vi "Test Q factor retrieval.vi"() -> ()   [LabVIEW 2012]
uses:
  Reusable/General/Math Utilities.lvlib
  <vilib>/Analysis/NI_AALBase.lvlib
  <vilib>/Analysis/baseanly.llb/Mean (DBL).vi
panel:
  out "Waveform Graph":dbl[][](graph)
  out "element":timestamp
  in  "Cell":i32
  out "Q with offset":dbl
  out "best fit parameters 2":dbl[](array[numeric])
  out "Q Factor 2":dbl
  in  "index":i32 min=0 max=1000
  out "prev Qfactor":dbl
  out "Q Factor":dbl
  out "best fit parameters":dbl[](array[numeric])
  in  "high":i32
  in  "low":i32
  out "XY Graph":cluster{i32[], "best fit parameters":dbl[]}[](graph)
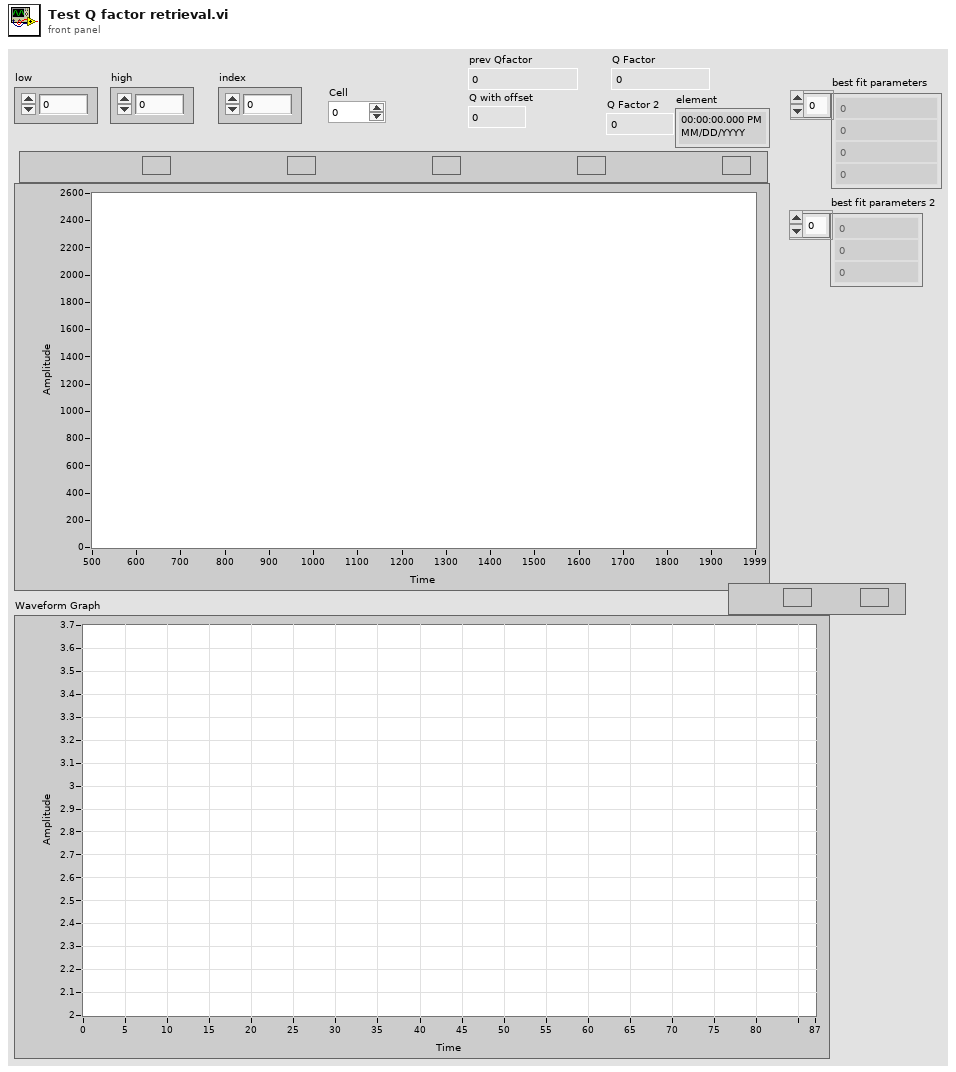
[diagram p1: front panel]
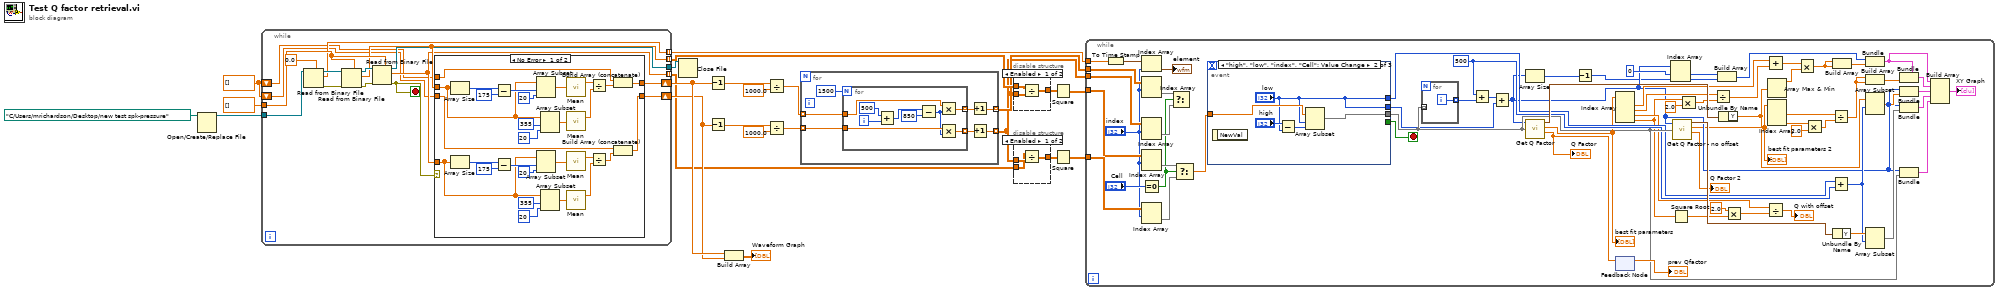
[diagram p0: block diagram]
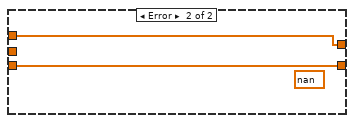
[diagram p4: hidden frame]
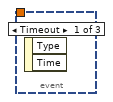
[diagram p5: hidden frame]
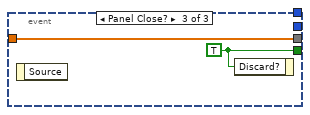
[diagram p6: hidden frame]
diagram:
  w18 = dbl[] []
  n1 = Open/Create/Replace File(file path (use dialog)=path "C:/Users/mrichardson/Desktop/new test spk-pressure") -> (refnum out=w23:refnum<file>)  [unwired: 5 in, 2 out]
  n2 = while {
    tunnel: w23 -> [w32]
    tunnel: dbl[] [] -> [w36]
    tunnel: [w39] -> w21
    tunnel: [w29] -> w1 mode=indexing
    tunnel: [w30] -> w6 mode=indexing
    tunnel: [w31] -> w19 mode=indexing
    shift-right: [w27] -> w16
    shift-left: w18 -> [w25]
    shift-right: [w26] -> w10
    shift-left: w18 -> [w24]
    stop <- w28 stop-if-true
    n3 = Read from Binary File(5:0.0, 11:w32) -> (0:w33:errorcluster, 2:w31:dbl, 3:w34:refnum<file>)  [unwired: 4 in, 1 out]
    n4 = Read from Binary File(5:w36, 8:w33, 11:w34) -> (0:w38:errorcluster, 2:w30:dbl[], 3:w37:refnum<file>)  [unwired: 3 in, 1 out]
    n5 = Read from Binary File(5:w36, 8:w38, 11:w37) -> (0:w28:errorcluster, 2:w29:dbl[], 3:w39:refnum<file>)  [unwired: 3 in, 1 out]
    n6 = case shown="No Error" w28 {
      tunnel: w30 -> [w63 _]
      tunnel: w29 -> [w41 _]
      tunnel: [w46 w69] -> w27
      tunnel: [w44 w68] -> w26
      tunnel: w25 -> [w43 w69]
      tunnel: w24 -> [w42 w68]
      frame No Error {
        n7 = Array Size(array=w63) -> (size(s)=w67:i32)
        n8 = Array Size(array=w41) -> (size(s)=w57:i32)
        n9 = Subtract(x=w67, y=175) -> (x-y=w65:i32)
        n10 = Subtract(x=w57, y=175) -> (x-y=w55:i32)
        n11 = Array Subset(array=w63, index=w65, length=20) -> (w59:dbl[])
        n12 = Array Subset(array=w41, index=w55, length=20) -> (w48:dbl[])
        n13 = Array Subset(array=w63, index=355, length=20) -> (w60:dbl[])
        n14 = Array Subset(array=w41, index=355, length=20) -> (w51:dbl[])
        n15 = call-poly <vilib>:"Mean.vi"("X"=w59) -> ("mean"=w40:dbl)  [unwired: 1 out]
        n16 = call-poly <vilib>:"Mean.vi"("X"=w60) -> ("mean"=w58:dbl)  [unwired: 1 out]
        n17 = call-poly <vilib>:"Mean.vi"("X"=w48) -> ("mean"=w50:dbl)  [unwired: 1 out]
        n18 = call-poly <vilib>:"Mean.vi"("X"=w51) -> ("mean"=w49:dbl)  [unwired: 1 out]
        n19 = Divide(x=w40, y=w58) -> (x/y=w47:dbl)
        n20 = Divide(x=w50, y=w49) -> (x/y=w45:dbl)
        n21 = Build Array (concatenate)(w43, w47) -> (w46:dbl[])
        n22 = Build Array (concatenate)(w42, w45) -> (w44:dbl[])
      }
      frame Error {
        (unwired) nan ("mean")
      }
    }
  }
  n23 = Close File(refnum=w21) -> ()  [unwired: 1 in, 2 out]
  n24 = Decrement(x=w16) -> (x-1=w15:dbl[])
  n25 = Decrement(x=w10) -> (x-1=w9:dbl[])
  n26 = Build Array(w16, w10) -> (→"Waveform Graph":dbl[][])
  n27 = Divide(x=w15, y=1000.0) -> (x/y=w12:dbl[])
  n28 = Divide(x=w9, y=1000.0) -> (x/y=w11:dbl[])
  n29 = for {
    tunnel: w12 -> [w75] mode=indexing
    tunnel: w11 -> [w76] mode=indexing
    tunnel: [w73] -> w4 mode=indexing
    tunnel: [w71] -> w3 mode=indexing
    n30 = for {
      N: 1500 -> [_]
      tunnel: w76 -> [w85]
      tunnel: w75 -> [w84]
      tunnel: [w83] -> w74 mode=indexing
      tunnel: [w82] -> w72 mode=indexing
      i -> [w81]
      n31 = Add(x=500, y=w81) -> (x+y=w79:i32)
      n32 = Subtract(x=w79, y=850) -> (x-y=w77:i32)
      n33 = Multiply(x=w84, y=w77) -> (x*y=w83:dbl)
      n34 = Multiply(x=w85, y=w77) -> (x*y=w82:dbl)
    }
    n35 = Increment(x=w74) -> (x+1=w73:dbl[])
    n36 = Increment(x=w72) -> (x+1=w71:dbl[])
  }
  n37 = disable-structure shown="Enabled" {
    disable-tunnel: w6 -> [w88 w89]
    disable-tunnel: [w87 w89] -> w5
    disable-tunnel: w4 -> [w86 _]
    frame Enabled {
      n38 = Divide(x=w88, y=w86) -> (x/y=w87:dbl[][])
    }
    frame Disabled {
    }
  }
  n39 = disable-structure shown="Enabled" {
    disable-tunnel: w3 -> [w92 _]
    disable-tunnel: w1 -> [w91 w93]
    disable-tunnel: [w90 w93] -> w2
    frame Enabled {
      n40 = Divide(x=w91, y=w92) -> (x/y=w90:dbl[][])
    }
    frame Disabled {
    }
  }
  n41 = Square(x=w5) -> (x^2=w8:dbl[][])
  n42 = Square(x=w2) -> (x^2=w7:dbl[][])
  n43 = while {
    tunnel: w7 -> [w153]
    tunnel: w8 -> [w107]
    tunnel: w19 -> [w103]
    tunnel: w4 -> [w100]
    tunnel: w3 -> [w99]
    stop <- w161 stop-if-true
    w145 = 500
    n44 = To Time Stamp(1:w103) -> (0:w102:timestamp[])
    n45 = Index Array(array=w102, index="index") -> (element=→"element":timestamp)
    n46 = Index Array(array=w100, index (row)="index") -> (element=w96:dbl[])  [unwired: 1 in]
    n47 = Index Array(array=w99, index (row)="index") -> (element=w97:dbl[])  [unwired: 1 in]
    n48 = Index Array(array=w107, index (row)="index") -> (element=w105:dbl[])  [unwired: 1 in]
    n49 = Equal To 0?(x="Cell") -> (x = 0?=w95:bool)
    n50 = Index Array(array=w153, index (row)="index") -> (element=w104:dbl[])  [unwired: 1 in]
    n51 = Select(t=w96, s=w95, f=w97) -> ()  [unwired: 1 out]
    n52 = Select(t=w105, s=w95, f=w104) -> (s? t:f=w94:dbl[])
    n53 = event shown="[1] \"high\", \"low\", \"index\", \"Cell\": Value Change" {
      selector: _ -> [_ _ _]
      dyn-events: _ -> [_ _ _]
      timeout: _ -> [_ _ _]
      tunnel: [_ _ w168] -> w161
      tunnel: w94 -> [_ w166 w169]
      tunnel: [_ w165 w169] -> w152
      tunnel: [_ "low" _] -> w146
      tunnel: [_ "low" _] -> w144
      event Timeout {
        n54 = event-data() -> ()  [unwired: 1 in, 2 out]
      }
      event "high", "low", "index", "Cell": Value Change {
        n55 = event-data() -> ()  [unwired: 1 in, 1 out]
        n56 = Subtract(x="high", y="low") -> (x-y=w164:i32)
        n57 = Array Subset(array=w166, index="low", length=w164) -> (w165:dbl[])
      }
      event Panel Close? {
        w168 = TRUE
        n58 = event-data() -> ()  [unwired: 1 in, 1 out]
        n59 = event-data("Discard?"=w168) -> ()  [unwired: 1 in, 1 out]
      }
    }
    n60 = for {
      tunnel: w152 -> [_] mode=indexing
      tunnel: [w162] -> w157 mode=indexing
      i -> [w162]
    }
    n61 = Add(x=w145, y=w157) -> (x+y=w147:i32[])
    n62 = Add(x=w147, y=w146) -> (x+y=w127:i32[])
    n63 = Array Size(array=w127) -> (size(s)=w126:i32)
    n64 = call "Get Q Factor.vi"("X"=w127, "Y"=w152) -> ("Fitted Data"=w160:waveform(dbl), "best fit parameters"=w142:dbl[], "Q Factor"=w159:dbl)  [unwired: 1 in, 2 out]
    "best fit parameters" <- w142
    "Q Factor" <- w159
    n65 = Decrement(x=w126) -> (x-1=w125:i32)
    n66 = Index Array(array=w142) -> (element #1=w129:dbl, element #2=w134:dbl, element #3=w138:dbl, element #4=w133:dbl)  [unwired: 4 in]
    n67 = feedback-in #1(w159) -> ()
    n68 = feedback #1() -> (→"prev Qfactor":dbl)  [unwired: 1 in]
    n69 = Index Array(array=w127, index #1=0 ("index"), index #2=w125) -> (element #1=w124:i32, element #2=w123:i32)
    n70 = Square Root(x=w133) -> (sqrt(x)=w141:dbl)
    n71 = call "Get Q Factor - no offset.vi"("X"=w127, "Y"=w152) -> ("Fitted Data"=w151:waveform(dbl), "best fit parameters"=w120:dbl[], "Q Factor"=→"Q Factor 2":dbl)  [unwired: 1 in, 2 out]
    "best fit parameters 2" <- w120
    n72 = Multiply(x=w133, y=2.0) -> (x*y=w131:dbl)
    n73 = Divide(x=w134, y=w131) -> (x/y=w130:dbl)
    n74 = Build Array(w124, w123) -> (w122:i32[])
    n75 = Unbundle By Name(w160) -> ("Y"=w111:dbl[])
    n76 = Multiply(x=2.0, y=w141) -> (x*y=w139:dbl)
    n77 = Add(x=w129, y=w130) -> (x+y=w110:dbl)
    n78 = Divide(x=w138, y=w139) -> (x/y=→"Q with offset":dbl)
    n79 = Array Max & Min(array=w111) -> (max value=w109:dbl)  [unwired: 3 out]
    n80 = Index Array(array=w120) -> (element #1=w116:dbl, element #3=w118:dbl)  [unwired: 3 in, 1 out]
    n81 = Multiply(x=w110, y=w109) -> (x*y=w108:dbl)
    n82 = Multiply(x=w118, y=2.0) -> (x*y=w117:dbl)
    n83 = Divide(x=w116, y=w117) -> (x/y=w115:dbl)
    n84 = Add(x=w144, y=w145) -> (x+y=w143:i32)
    n85 = Build Array(w108, w108) -> (w121:dbl[])
    n86 = Unbundle By Name(w151) -> ("Y"=w150:dbl[])
    n87 = Bundle(w122, w121) -> (w113:cluster{i32[], dbl[]})  [unwired: 1 in]
    n88 = Build Array(w115, w115) -> (w114:dbl[])
    n89 = Array Subset(array=w111, index=w143) -> (w154:dbl[])  [unwired: 1 in]
    n90 = Array Subset(array=w150, index=w143) -> (w149:dbl[])  [unwired: 1 in]
    n91 = Bundle(cluster=w113, w114) -> (w112:cluster{i32[], dbl[]})  [unwired: 1 in]
    n92 = Bundle(w127, w154) -> (w156:cluster{i32[], dbl[]})  [unwired: 1 in]
    n93 = Bundle(w127, w149) -> (w135:cluster{i32[], dbl[]})  [unwired: 1 in]
    n94 = Bundle(w127, w152) -> (w136:cluster{i32[], dbl[]})  [unwired: 1 in]
    n95 = Build Array(w113, w112, w156, w135, w136) -> (→"XY Graph":cluster{i32[], dbl[]}[])
  }
